vi "Sub Initialize.vi"(8 "error in (no error)":errorcluster, 11 "Instrument Recorder in":refnum<class "RP Delayed.lvclass">) -> (0 "error out":errorcluster, 2 "Initialize Result":refnum<class "Acquired Result.lvclass">, 3 "Instrument Recorder out":refnum<class "RP Delayed.lvclass">)   [LabVIEW 2016, in "RP Delayed.lvclass"]
uses:
  RP Delayed.lvclass
  C:/github/LabActor/Pulse Recorders/Pulse Recorder/Pulse Recorder.lvclass
  C:/github/LabActor/Template Module/Template Module.lvclass
  NHMFL_Core/Libraries/Instruments/Results/Acquired Result/Acquired Result.lvclass
  NHMFL_Core/Libraries/Red Pitaya/Red Pitaya Digitizer/Red Pitaya Digitizer.lvclass
  C:/github/NHMFL_Core/Libraries/Instruments/Pulse Driver/Pulse Driver.lvclass
  Template Module/Template Module.lvclass/Template Module.ctl
  Template Module/Write Configuration.vi
  Pulse Recorders/Pulse Recorder/Read Pulse driver.vi
  Pulse Recorders/Pulse Recorder/Write Pulse driver.vi
  NHMFL_Core/Libraries/Instruments/Pulse Driver/Pulse Driver.lvclass
  Pulse Recorders/Pulse Recorder/Pulse Recorder.lvclass
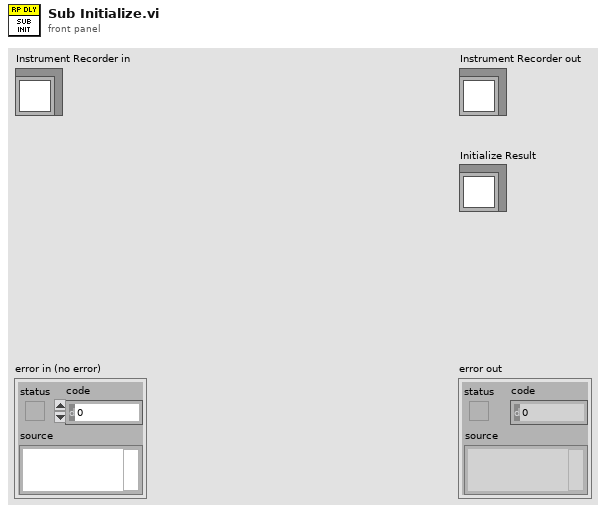
[diagram p1: front panel]
types:
  T1 = typedef "RP Delayed Configuration.ctl" = cluster{"Pre-trigger duration":dbl, "Post-trigger duration":dbl, "Rate":dbl, "Ranges":dbl[], "Re-name channels":string[], "Active channels":string, "External clock":bool, "Output delay":dbl, "After delay":bool}
  T2 = typedef "Pusle Driver Configuration.ctl" = cluster{"Pre-trigger duration":dbl, "Post-trigger duration":dbl, "Rate":dbl, "Ranges":dbl[], "Re-name channels":string[], "Active channels":string, "External clock":bool}
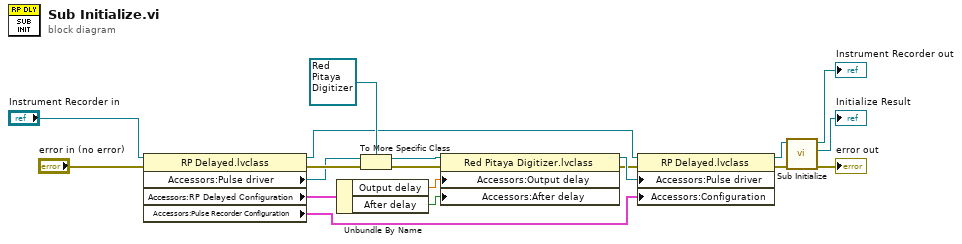
[diagram p0: block diagram]
diagram:
  n1 = property class="RP Delayed.lvclass"(reference="Instrument Recorder in", error in="error in (no error)") -> (reference out=w7:refnum<class "RP Delayed.lvclass">, error out=w16:errorcluster, "Accessors:Pulse driver"=w15:refnum<class "Pulse Driver.lvclass">, "Accessors:RP Delayed Configuration"=w12:T1, "Accessors:Pulse Recorder Configuration"=w2:T2)
  n2 = Unbundle By Name(w12) -> ("Output delay"=w11:dbl, "After delay"=w1:bool)
  n3 = To More Specific Class(target class=refnum<class "Red Pitaya Digitizer.lvclass"> refnum ("Red Pitaya Digitizer.lvclass"), reference=w15, error in=w16) -> (specific class reference=w13:refnum<class "Red Pitaya Digitizer.lvclass">, error out=w10:errorcluster)
  n4 = property class="Red Pitaya Digitizer.lvclass"(reference=w13, error in=w10, "Accessors:Output delay"=w11, "Accessors:After delay"=w1) -> (reference out=w9:refnum<class "Red Pitaya Digitizer.lvclass">, error out=w6:errorcluster)
  n5 = property class="RP Delayed.lvclass"(reference=w7, error in=w6, "Accessors:Pulse driver"=w9, "Accessors:Configuration"=w2) -> (reference out=w3:refnum<class "RP Delayed.lvclass">, error out=w4:errorcluster)
  n6 = call-parent "Sub Initialize.vi"("error in (no error)"=w4, "Instrument Recorder in"=w3) -> ("error out"=→"error out":errorcluster, "Initialize Result"=→"Initialize Result":refnum<class "Acquired Result.lvclass">, "Instrument Recorder out"=→"Instrument Recorder out":refnum<class "RP Delayed.lvclass">)  [unwired: 7 in]
